vi "Generate PPS-cRIO9039(FPGA).vi"() -> ()   [LabVIEW 2016]
uses:
  <vilib>/Platform/TimedLoop/XDataNode/timing_clust.ctl
  <vilib>/Platform/TimedLoop/XDataNode/nitl_modes.ctl
  <vilib>/Platform/TimedLoop/XDataNode/wakeup.ctl
  <vilib>/rvi/eio/common/nirviEmuTemplateMethod_errors.vi
  <vilib>/rvi/Emulation/niFpgaSctlEmulationGetInTimedLoop.vi
  <vilib>/rvi/Emulation/niFpgaEmulationReportErrorSimple.vi
  <vilib>/rvi/Emulation/niFpgaGetClockAttributes.vi
  <vilib>/rvi/Emulation/niFpgaCriticalErrorInLSC.vi
  <instrlib>/_niInstr/Basic Elements/v1/FPGA/Private/Count Up U64.vi
  <vilib>/eio/EIOMethodNode/EIOMethodNode.xnode
  <vilib>/Platform/TimedLoop/XDataNode/XDataNode.xnode
  <vilib>/eio/EIONode/EIONode.xnode
  <vilib>/Platform/TimedLoop/XDataNode/XDNodeRunTimeDep.lvlib
  <instrlib>/_niInstr/Basic Elements/v1/FPGA/niInstr Basic Elements v1 FPGA.lvlib
panel:
  out "Current Time":u64
  in  "PulseWidth(Ticks)":u64 format="%.0p"
  in  "Start Time":u64
  out "NumPulses Sentout":u64
  out "Offset from Time Reference":i32
  out "Offset from Time Reference Valid":bool
  out "Sync Epoch":bool
  out "Time Synchronization Fault":bool
  out "Time Source":enum8{"None", "System", "External"}(ring)
  in  "Tx Pulse Ticks":u64=40000 format="%.0p"
  out "PPS Counter":u64 format="%.0p"
  in  "DIO3_Enable":bool=TRUE
  in  "DIO2_Enable":bool=TRUE
  in  "DIO1_Enable":bool=TRUE
  in  "DIO0_Enable":bool=TRUE
  # "Tx Pulse Ticks shouldn't be changed\nrun-time on FPGA (prefe 40k)"
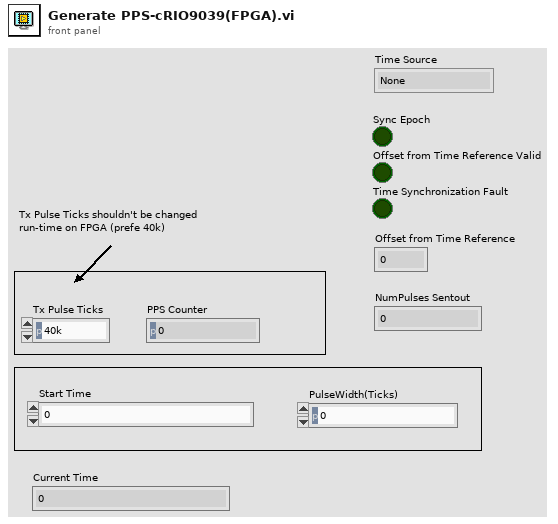
[diagram p1: front panel]
types:
  T1 = typedef "XDNodeRunTimeDep.lvlib/timing_clust.ctl" = cluster{"Expected End [f-1]":u64, "Actual End [f-1]":u64, "Finished Late? [f-1]":bool, "Expected End [i-1]":u64, "Actual End [i-1]":u64, "Finished Late? [i-1]":bool, "Expected Start [i]":u64, "Actual Start [i]":u64, "Expected Start [f]":u64, "Actual Start [f]":u64, "Source Name":string, "Structure Name":string, "Period":i64, "Deadline":i64, "Offset":i64, "Start":i64, "Priority":i32, "Timeout":i32, "Mode":T2, "Wakeup Reason":T3, "Error":errorcluster, "Source Type":string, "Secondary Source Type":string, "Global End Time":u64, "Global Start Time":u64, "Frame Duration":u64, "Iteration Duration":u64, "Assigned CPU":i32, "I/O Scan Engine Mode":u32}
  T2 = typedef "XDNodeRunTimeDep.lvlib/nitl_modes.ctl" = enum32{"No Change", "Process missed periods, maintain original phase", "Discard missed periods, maintain original phase", "Process missed periods, ignore original phase", "Discard missed periods, ignore original phase"}
  T3 = typedef "XDNodeRunTimeDep.lvlib/wakeup.ctl" = enum32{"Normal", "Aborted", "Asynchronous wakeup", "Timing source error", "Timed loop error", "Timeout"}
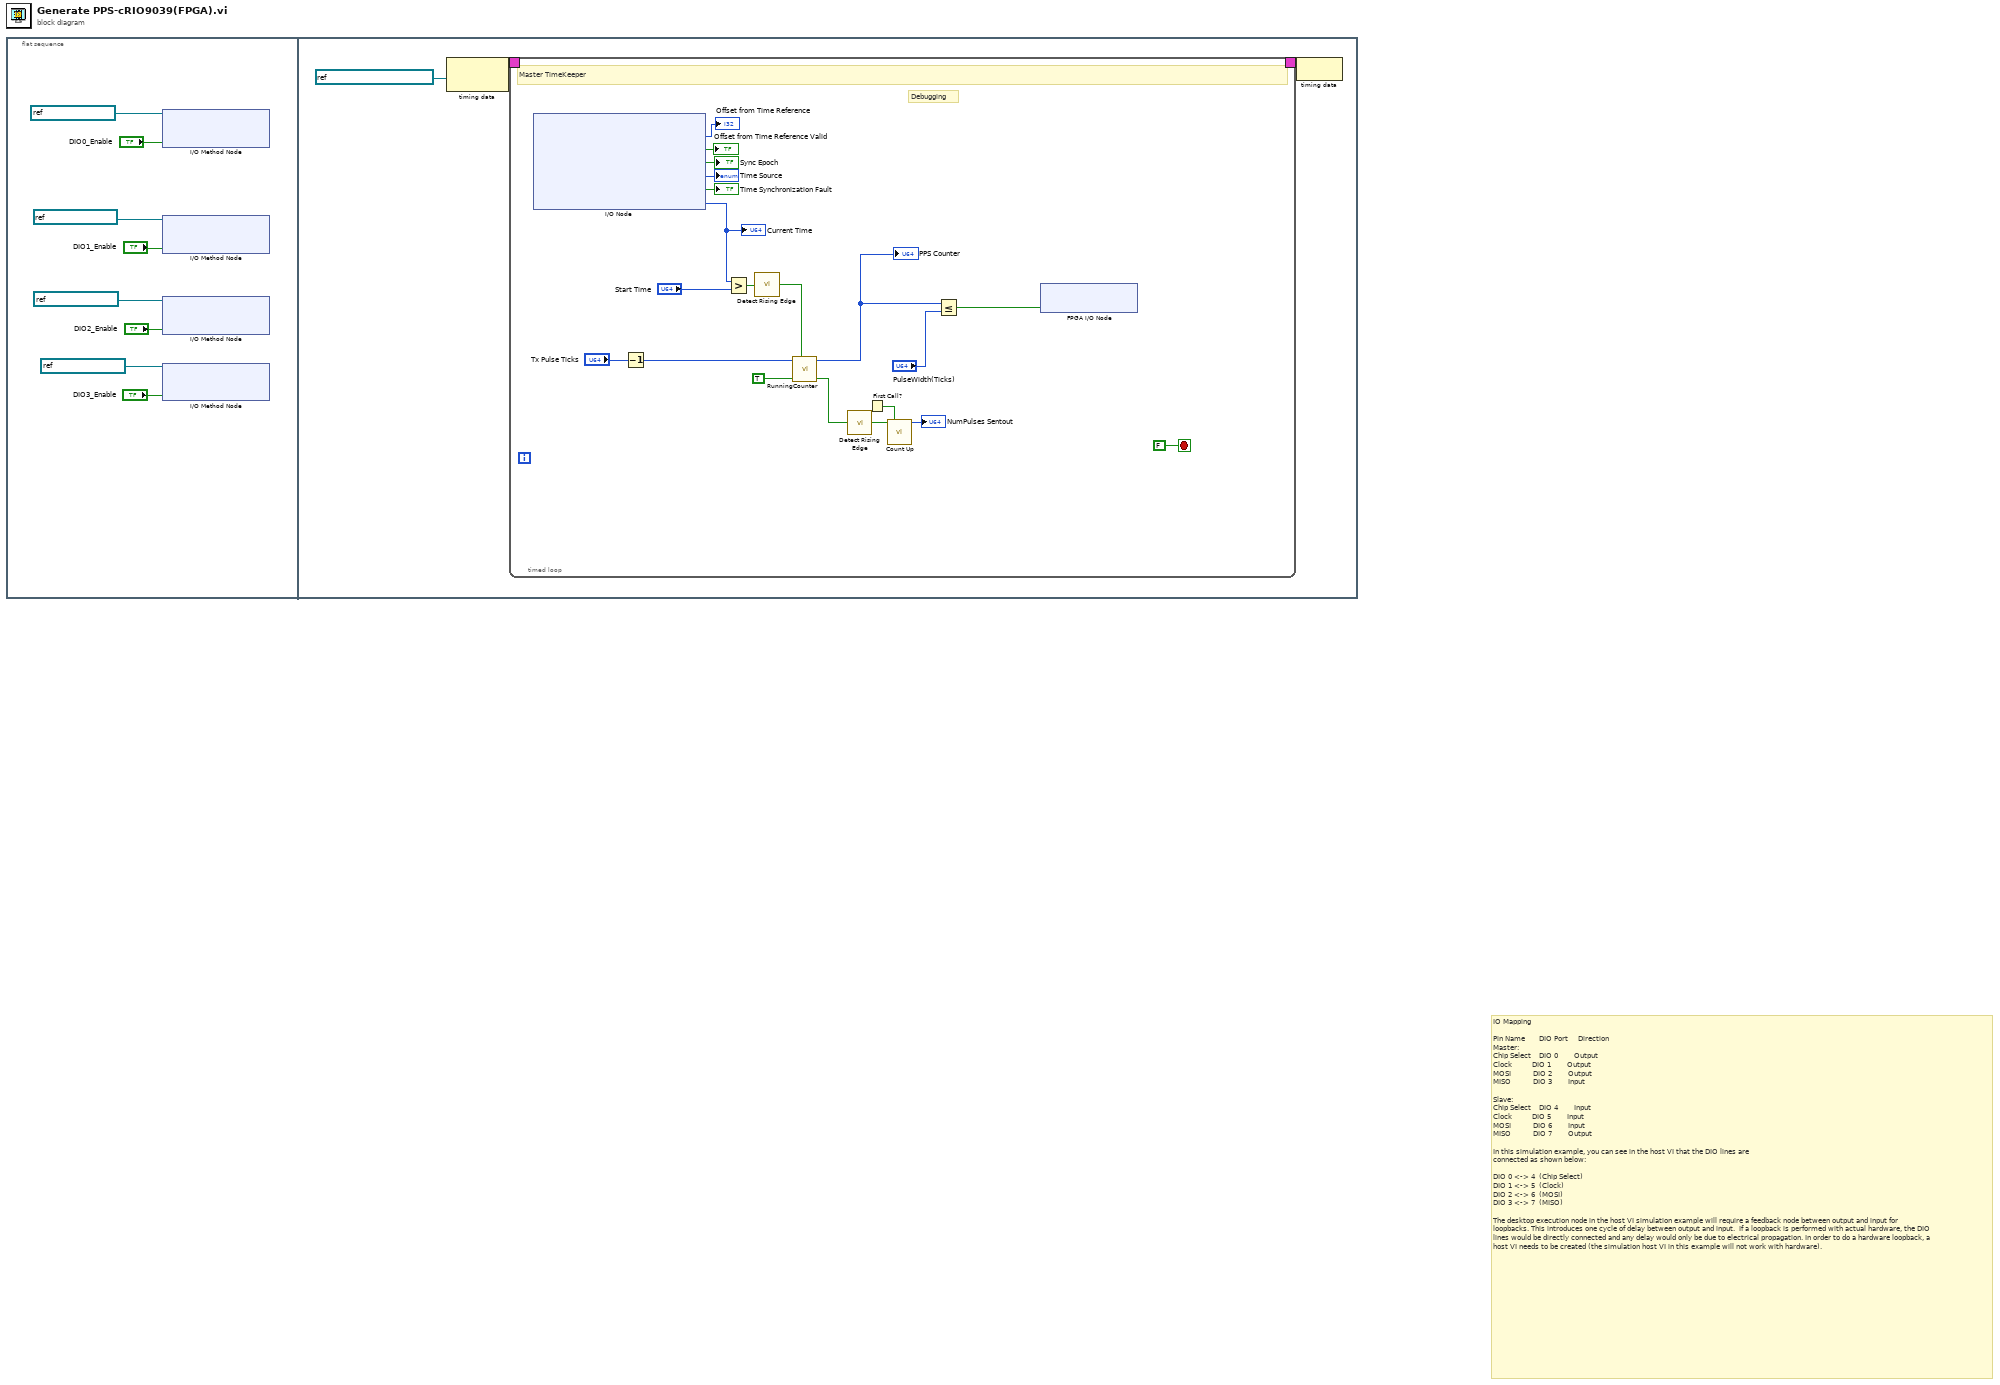
[diagram p0: block diagram]
diagram:
  # "IO Mapping\n\nPin Name       DIO Port     Direction        \nMaster: \nChip Select    DIO 0        Output           \nClock          DIO 1        Output           \nMOSI           DIO 2        Output           \nMISO           DIO 3        Input            \n\nSlave:\nChip Select    DIO 4        Input            \nClock          DIO 5        Input            \nMOSI           DIO 6        Input            \nMISO           DIO 7        Output           \n\nIn this simulation example, you can see in the host VI that the DIO lines are\nconnected as shown below:\n\nDIO 0 <-> 4  (Chip Select)\nDIO 1 <-> 5  (Clock)\nDIO 2 <-> 6  (MOSI)\nDIO 3 <-> 7  (MISO)\n\nThe desktop execution node in the host VI simulation example will require a feedback node between output and input for loopbacks. This introduces one cycle of delay between output and input.  If a loopback is performed with actual hardware, the DIO lines would be directly connected and any delay would only be due to electrical propagation. In order to do a hardware loopback, a host VI needs to be created (the simulation host VI in this example will not work with hardware)."
  n1 = flat-sequence {
    frame #0 {
      n2 = xnode "I/O Method Node"("FPGA I/O In"=refnum<k21> "Mod9402/DIO0", "Enable"="DIO0_Enable") -> ()  [unwired: 1 out]
      n3 = xnode "I/O Method Node"("FPGA I/O In"=refnum<k21> "Mod9402/DIO1", "Enable"="DIO1_Enable") -> ()  [unwired: 1 out]
      n4 = xnode "I/O Method Node"("FPGA I/O In"=refnum<k21> "Mod9402/DIO2", "Enable"="DIO2_Enable") -> ()  [unwired: 1 out]
      n5 = xnode "I/O Method Node"("FPGA I/O In"=refnum<k21> "Mod9402/DIO3", "Enable"="DIO3_Enable") -> ()  [unwired: 1 out]
    }
    frame #1 {
      n6 = node-c288(refnum<k21> "40 MHz Onboard Clock" ("Source Name")) -> (w11:T1)
      n7 = timed-loop "SPI Master Interface" {
        timing: w11 -> [_]
        timing-out: [_] -> w10
        stop <- FALSE stop-if-true
        # "Debugging"
        # "Master TimeKeeper"
        n8 = xnode "I/O Node"() -> ("Offset from Time Reference"=→"Offset from Time Reference":i32, "Offset from Time Reference Valid"=→"Offset from Time Reference Valid":bool, "Sync Epoch"=→"Sync Epoch":bool, "Time Source"=→"Time Source":enum8{"None", "System", "External"}, "Time Synchronization Fault"=→"Time Synchronization Fault":bool, "Time"=w19:u64)  [unwired: 6 in, 6 out]
        "Current Time" <- w19
        n9 = Decrement(x="Tx Pulse Ticks") -> (x-1=w20:u64)
        n10 = Greater?(x=w19, y="Start Time") -> (0:w17:bool)
        n11 = call <instrlib>:"Detect Rising Edge.vi"("signal"=w17) -> ("edge detected"=w16:bool)  [unwired: 14 in]
        n12 = call "RunningCounter.vi"("Reset?"=w16, "INC?"=TRUE, "rollover"=w20) -> ("rollover"=w15:bool, "count"=w14:u64)  [unwired: 7 in]
        "PPS Counter" <- w14
        n13 = call <instrlib>:"Detect Rising Edge.vi"("signal"=w15) -> ("edge detected"=w23:bool)  [unwired: 14 in]
        n14 = First Call?() -> (First Call?: T/F=w21:bool)
        n15 = call-poly <instrlib>:"Count Up.vi"("increment"=w23, "reset"=w21) -> ("count out"=→"NumPulses Sentout":u64)  [unwired: 13 in]
        n16 = Less Or Equal?(x=w14, y="PulseWidth(Ticks)") -> (x <= y?=w12:bool)
        n17 = xnode "FPGA I/O Node"("Mod9402/DIO0"=w12) -> ()  [unwired: 1 in, 1 out]
      }
      n18 = node-c288(w10) -> ()
    }
  }
